vi "Save NIC Settings.vi"(7 "Network Interface:":u16, 8 "Error In":errorcluster, 11 "Install LV Data":T1) -> (0 "Error Out":errorcluster, 3 "Install LV Data":T1)   [LabVIEW 2020, in "LMH-LINX.lvlib"]
uses:
  LMH-LINX.lvlib
  Install LV Data.ctl
  Target Info.ctl
  NIC Info.ctl
  NIC Mode.ctl
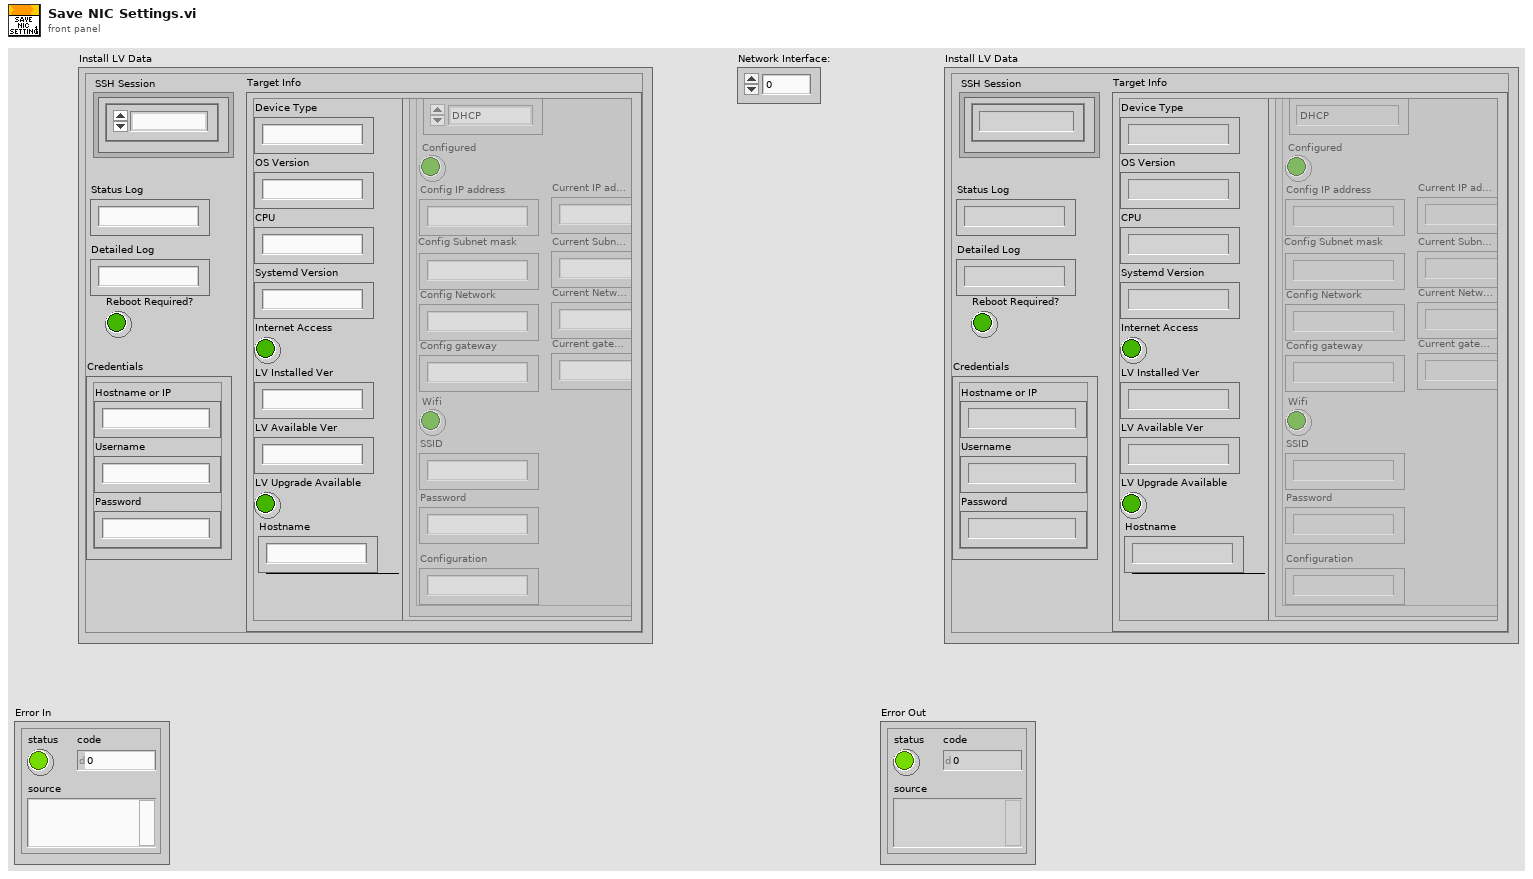
[diagram p1: front panel]
types:
  T1 = typedef "LMH-LINX.lvlib/Install LV Data.ctl" = cluster{"SSH Session":refnum<k1>, "Status Log":string, "Detailed Log":string, "Credentials":cluster{"Hostname or IP":string, "Username":string, "Password":string}, "Target Info":T2, "Reboot Required?":bool}
  T2 = typedef "LMH-LINX.lvlib/Target Info.ctl" = cluster{"OS Version":string, "CPU":string, "Systemd Version":string, "Internet Access":bool, "Device Type":string, "LV Installed Ver":string, "LV Available Ver":string, "LV Upgrade Available":bool, "Hostname":string, "NIC Info":T3[]}
  T3 = typedef "LMH-LINX.lvlib/NIC Info.ctl" = cluster{"Name":string, "NIC Mode":T4, "Configured":bool, "Config IP address":string, "Config Subnet mask":string, "Config Network":string, "Config gateway":string, "Wifi":bool, "SSID":string, "Password":string, "Configuration":string, "Current IP address":string, "Current Subnet mask":string, "Current gateway":string, "Current Network":string}
  T4 = typedef "LMH-LINX.lvlib/NIC Mode.ctl" = enum16{"DHCP", "Static", "Loopback"}
  T5 = typedef "LMH-LINX.lvlib/Network Settings Ctrl Refs.ctl" = cluster{"Hostname":refnum<vi>, "IP address":refnum<vi>, "Subnet mask":refnum<vi>, "Default Gateway":refnum<vi>, "SSID":refnum<vi>, "Password":refnum<vi>, "NIC Status":refnum<vi>, "Network Interface":refnum<vi>, "DCHP":refnum<vi>}
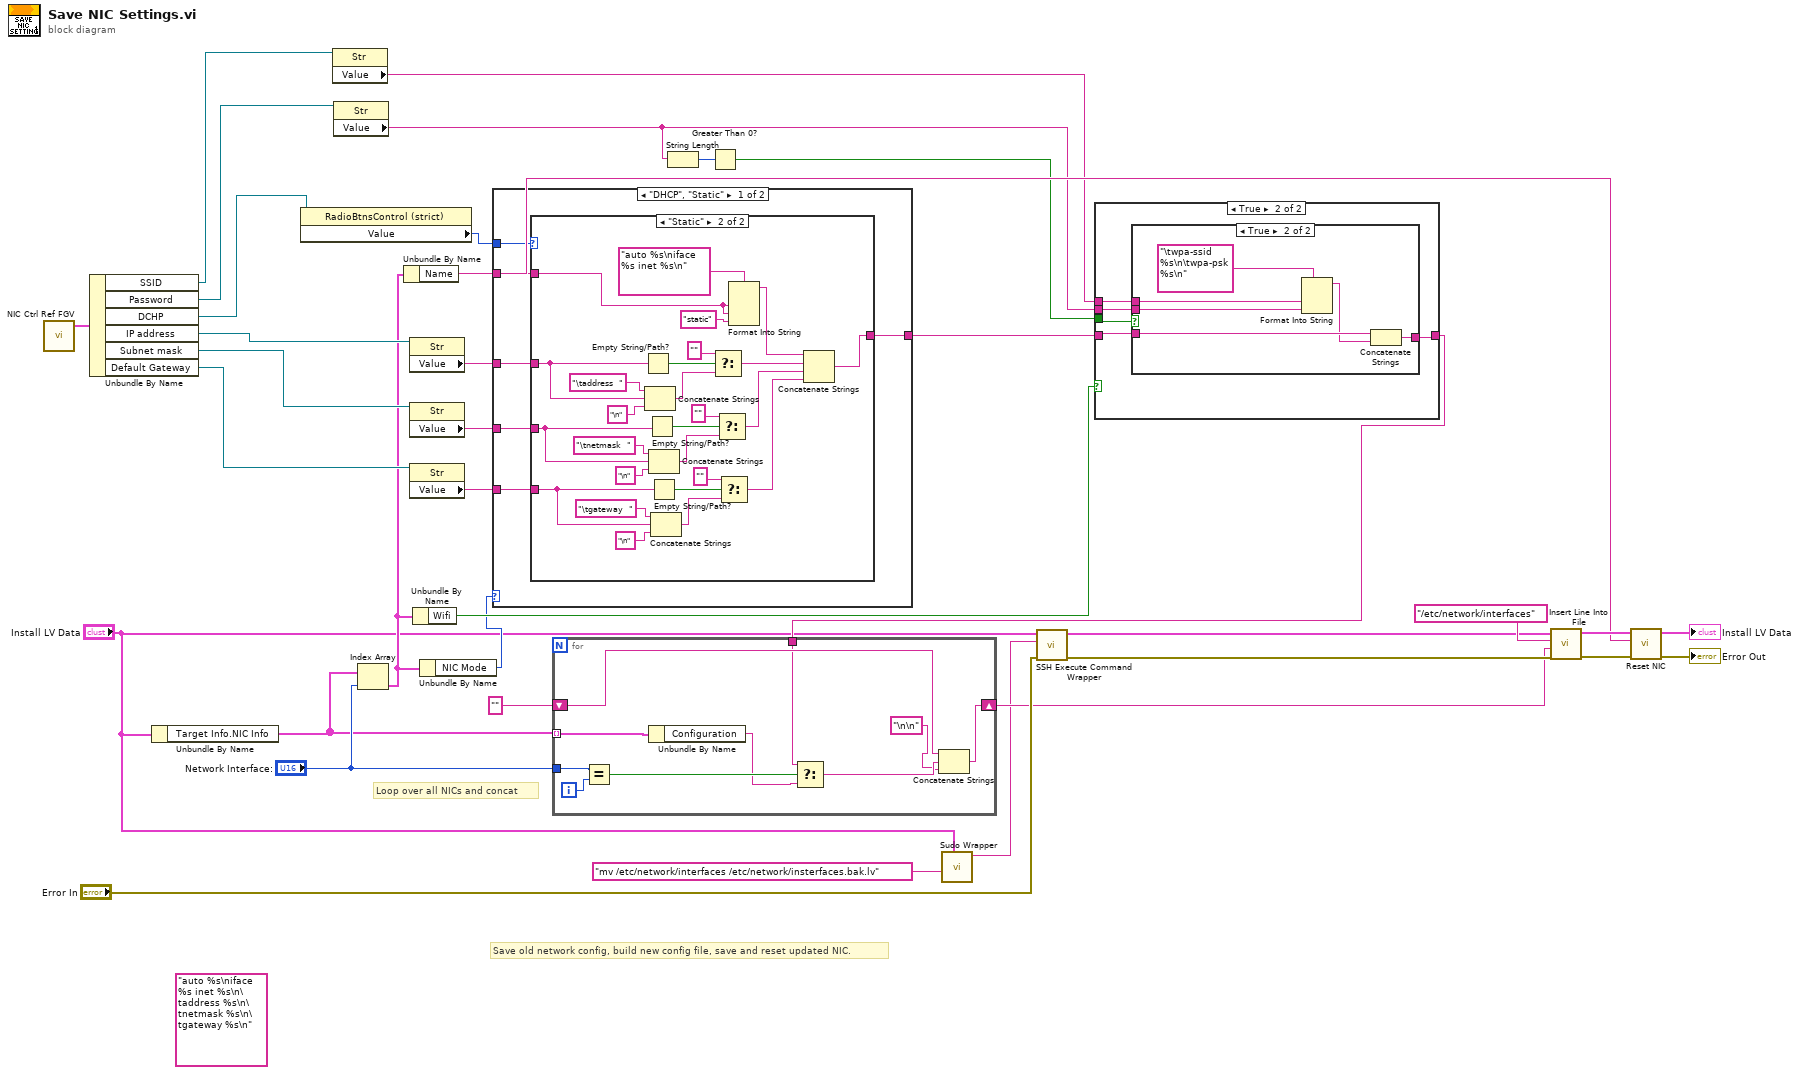
[diagram p0: block diagram]
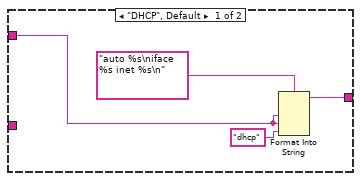
[diagram p2: hidden frame]
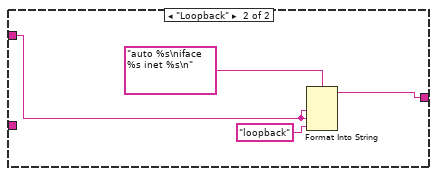
[diagram p3: hidden frame]
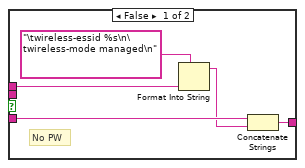
[diagram p5: hidden frame]
diagram:
  (unwired) "auto %s\niface %s inet %s\n\taddress %s\n\tnetmask %s\n\tgateway %s\n"
  # "Loop over all NICs and concat"
  # "Save old network config, build new config file, save and reset updated NIC."
  n1 = call "NIC Ctrl Ref FGV.vi"() -> ("Network Settings Ctrl Refs"=w28:T5)  [unwired: 4 in]
  n2 = Unbundle By Name(w28) -> ("SSID"=w21:refnum<vi>, "Password"=w20:refnum<vi>, "DCHP"=w29:refnum<vi>, "IP address"=w31:refnum<vi>, "Subnet mask"=w32:refnum<vi>, "Default Gateway"=w33:refnum<vi>)
  n3 = Unbundle By Name("Install LV Data") -> ("Target Info.NIC Info"=w11:T3[])
  n4 = property class="RadioBtnsControl (strict)"(reference=w29) -> ("Value"=w30:enum32{"DHCP", "Static"})  [unwired: 1 in, 2 out]
  n5 = property class="Str"(reference=w21) -> ("Value"=w19:string)  [unwired: 1 in, 2 out]
  n6 = property class="Str"(reference=w20) -> ("Value"=w18:string)  [unwired: 1 in, 2 out]
  n7 = Index Array(array=w11, index="Network Interface:") -> (element=w10:T3)
  n8 = Unbundle By Name(w10) -> ("Name"=w26:string)
  n9 = property class="Str"(reference=w31) -> ("Value"=w34:string)  [unwired: 1 in, 2 out]
  n10 = property class="Str"(reference=w32) -> ("Value"=w35:string)  [unwired: 1 in, 2 out]
  n11 = property class="Str"(reference=w33) -> ("Value"=w36:string)  [unwired: 1 in, 2 out]
  n12 = Unbundle By Name(w10) -> ("Wifi"=w13:bool)
  n13 = Unbundle By Name(w10) -> ("NIC Mode"=w9:T4)
  n14 = case shown="\"DHCP\", \"Static\"" w9 {
    tunnel: w36 -> [w42 _]
    tunnel: w35 -> [w41 _]
    tunnel: w34 -> [w40 _]
    tunnel: w30 -> [w39 _]
    tunnel: w26 -> [w38 w74]
    tunnel: [w37 w73] -> w22
    frame "DHCP", "Static" {
      n15 = case shown="\"Static\"" w39 {
        tunnel: [w44 w62] -> w37
        tunnel: w38 -> [w43 w70]
        tunnel: w40 -> [_ w65]
        tunnel: w41 -> [_ w53]
        tunnel: w42 -> [_ w52]
        frame "DHCP", Default {
          n16 = Format Into String(format string="auto %s\niface %s inet %s\n", w43, w43, "dhcp" ("input 2")) -> (resulting string=w44:string)  [unwired: 2 in, 1 out]
        }
        frame "Static" {
          n17 = Empty String/Path?(string/path=w65) -> (empty?=w67:bool)
          n18 = Concatenate Strings("\taddress  ", w65, "\n" ("string")) -> (w68:string)
          n19 = Empty String/Path?(string/path=w53) -> (empty?=w60:bool)
          n20 = Concatenate Strings("\tnetmask  ", w53, "\n" ("string")) -> (w59:string)
          n21 = Empty String/Path?(string/path=w52) -> (empty?=w55:bool)
          n22 = Concatenate Strings("\tgateway  ", w52, "\n" ("string")) -> (w56:string)
          n23 = Select(t="", s=w67, f=w68) -> (s? t:f=w63:string)
          n24 = Select(t="", s=w60, f=w59) -> (s? t:f=w51:string)
          n25 = Select(t="", s=w55, f=w56) -> (s? t:f=w50:string)
          n26 = Format Into String(format string="auto %s\niface %s inet %s\n", w70, w70, "static" ("input 2")) -> (resulting string=w64:string)  [unwired: 2 in, 1 out]
          n27 = Concatenate Strings(w64, w63, w51, w50) -> (w62:string)
        }
      }
    }
    frame "Loopback" {
      n28 = Format Into String(format string="auto %s\niface %s inet %s\n", w74, w74, "loopback" ("input 2")) -> (resulting string=w73:string)  [unwired: 2 in, 1 out]
    }
  }
  n29 = String Length(string=w18) -> (length=w17:i32)
  n30 = Greater Than 0?(x=w17) -> (x > 0?=w16:bool)
  n31 = call "Sudo Wrapper.vi"("Install LV Data"="Install LV Data", "comand string"="mv /etc/network/interfaces /etc/network/insterfaces.bak.lv" ("Command")) -> ("combined command string"=w2:string)  [unwired: 9 in]
  n32 = call "SSH Execute Command Wrapper.vi"("Error In"="Error In", "Command"=w2, "Install LV Data in"="Install LV Data") -> ("Error Out"=w7:errorcluster, "Install LV Data out"=w5:T1)  [unwired: 6 in, 1 out]
  n33 = case shown="True" w13 {
    tunnel: [w77 w81] -> w6
    tunnel: w22 -> [w77 w80]
    tunnel: w19 -> [_ w82]
    tunnel: w18 -> [_ w78]
    tunnel: w16 -> [_ w79]
    frame False {
      # "Not Wifi...Move Along..."
    }
    frame True {
      n34 = case shown="True" w79 {
        tunnel: w82 -> [w86 w93]
        tunnel: [w85 w92] -> w81
        tunnel: w80 -> [w84 w91]
        tunnel: w78 -> [_ w89]
        frame False {
          # "No PW"
          n35 = Format Into String(format string="\twireless-essid %s\n\twireless-mode managed\n", w86) -> (resulting string=w83:string)  [unwired: 2 in, 1 out]
          n36 = Concatenate Strings(w84, w83) -> (w85:string)
        }
        frame True {
          n37 = Format Into String(format string="\twpa-ssid %s\n\twpa-psk %s\n", w93, w89) -> (resulting string=w90:string)  [unwired: 2 in, 1 out]
          n38 = Concatenate Strings(w91, w90) -> (w92:string)
        }
      }
    }
  }
  n39 = for {
    tunnel: "Network Interface:" -> [w103]
    tunnel: w11 -> [w98] mode=indexing
    shift-right: [w101] -> w4
    shift-left: "" ("string") -> [w100]
    tunnel: w6 -> [w97]
    i -> [w102]
    n40 = Equal?(x=w103, y=w102) -> (x = y?=w99:bool)
    n41 = Unbundle By Name(w98) -> ("Configuration"=w96:string)
    n42 = Select(t=w97, s=w99, f=w96) -> (s? t:f=w95:string)
    n43 = Concatenate Strings(w100, w95, "\n\n" ("string")) -> (w101:string)
  }
  n44 = call "Insert Line Into File.vi"("Error In"=w7, "Line"=w4, "File Path"="/etc/network/interfaces", "Install LV Data"=w5) -> ("Error Out"=w25:errorcluster, "Install LV Data"=w27:T1)  [unwired: 4 in, 2 out]
  n45 = call "Reset NIC.vi"("Error In"=w25, "NIC Name"=w26, "Install LV Data"=w27) -> ("Error Out"=→"Error Out":errorcluster, "Install LV Data out"=→"Install LV Data":T1)  [unwired: 7 in]
